vi "Two Sensor Line Following.vi"(10 "Sensor Array":bool[](array[boolean]), 11 "Left or Straight":bool) -> (2 "Motor Values":dbl[](array[numeric]), 3 "Left or Straight End":bool)   [LabVIEW 2018]
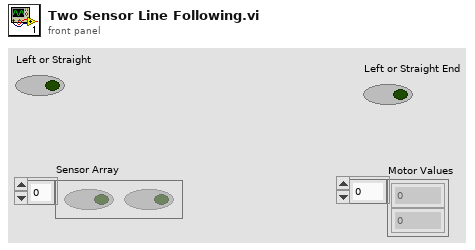
[diagram p1: front panel]
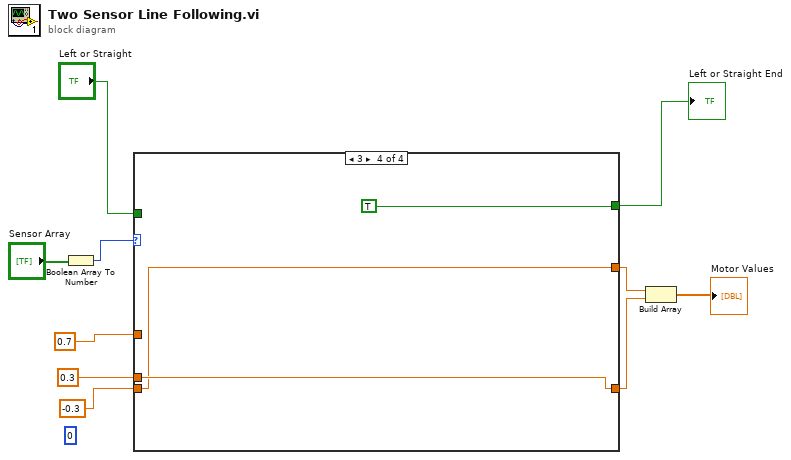
[diagram p0: block diagram]
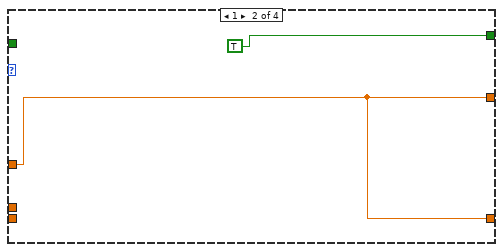
[diagram p4: hidden frame]
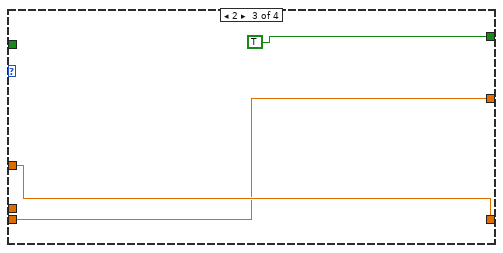
[diagram p5: hidden frame]
diagram:
  (unwired) 0
  n1 = Boolean Array To Number(Boolean array="Sensor Array") -> (number=w9:u32)
  n2 = case shown="3" w9 {
    tunnel: "Left or Straight" -> [w16 _ _ _]
    tunnel: 0.7 -> [w15 w24 w27 _]
    tunnel: [w14 w24 w26 w29] -> w5
    tunnel: -0.3 -> [w13 _ w26 w29]
    tunnel: [w12 w24 w27 w30] -> w4
    tunnel: 0.3 -> [_ _ _ w30]
    tunnel: [w11 TRUE TRUE TRUE] -> w2
    frame 0, Default {
      n3 = case shown="True" w16 {
        selector: w16 -> [w17 w20]
        tunnel: w15 -> [w19 w22]
        tunnel: [w18 w22] -> w14
        tunnel: [w19 w21] -> w12
        tunnel: w13 -> [w18 w21]
        tunnel: [w17 w20] -> w11
        frame False {
        }
        frame True {
        }
      }
    }
    frame 1 {
    }
    frame 2 {
    }
    frame 3 {
    }
  }
  "Left or Straight End" <- w2
  n4 = Build Array(w5, w4) -> (→"Motor Values":dbl[])
